vi "Evaluate Part 2.vi"() -> ()   [LabVIEW 2020]
uses:
  Game/Game.lvclass
  Bag/Bag.lvclass
panel:
  out "sum":i32=2286
  out "Powers":i32[](array[numeric])=[48, 12, 1560, 630, 36]
  in  "Input":string="Game 1: 3 blue, 4 red; 1 red, 2 green, 6 blue; 2 green\nGame 2: 1 blue, 2 green; 3 green, 4 blue, 1 red; 1 green, 1 blue\nGame 3: 8 green, 6 blue, 20 red; 5 blue, 4 red, 13 green; 5 green, 1 red\nGame 4: 1 green, 3 red, 6 blue; 3 green, 6 red; 3 green, 15 blue, 14 red\nGame 5: 6 red, 1 blue, 3 green; 2 blue, 1 red, 2 green"
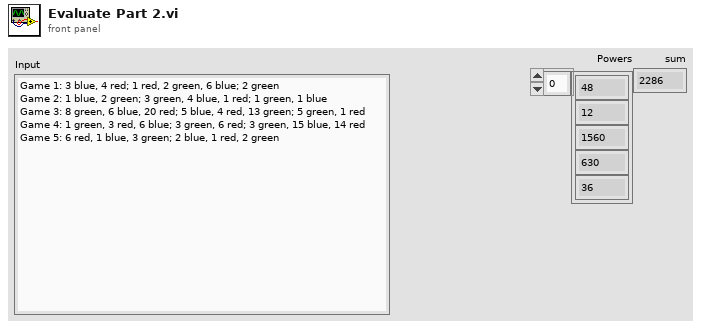
[diagram p1: front panel]
types:
  T1 = typedef "Bag.lvclass/Cubes.ctl" = cluster{"Red":i32, "Green":i32, "Blue":i32}
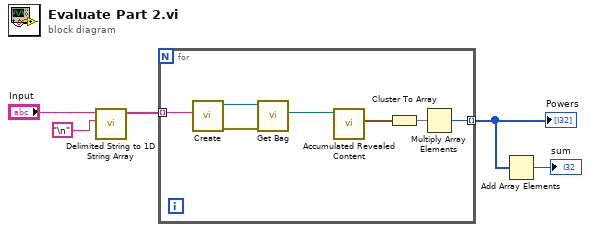
[diagram p0: block diagram]
diagram:
  n1 = call <vilib>:"Delimited String to 1D String Array.vi"("delimiter"="\n", "delimited string"="Input") -> ("string array"=w3:string[])  [unwired: 9 in]
  n2 = for {
    tunnel: w3 -> [w10] mode=indexing
    tunnel: [w6] -> w2 mode=indexing
    n3 = call "Create.vi"("Input"=w10) -> ("error out"=w11:errorcluster, "Game"=w12:refnum<class "Game.lvclass">)  [unwired: 9 in]
    n4 = call "Get Bag.vi"("error in (no error)"=w11, "Game in"=w12) -> ("Bag"=w9:refnum<class "Bag.lvclass">)  [unwired: 7 in, 2 out]
    n5 = call "Accumulated Revealed Content.vi"("Bag in"=w9) -> ("Cubes"=w8:T1)  [unwired: 8 in, 2 out]
    n6 = Cluster To Array(cluster=w8) -> (array=w7:i32[])
    n7 = Multiply Array Elements(1:w7) -> (0:w6:i32)
  }
  "Powers" <- w2
  n8 = Add Array Elements(numeric array=w2) -> (sum=→"sum":i32)
